vi "RedistributeArmPathPoints.vi"(1 "Desired Point Spacing (in)":dbl, 2 "Path Length (in)":dbl, 3 "ArmPathIn":T1[](array[typedef]), 4 "IndexedPathLength":dbl[](array[numeric])) -> (0 "ArmPathOut":T1[](array[typedef]))   [LabVIEW 2018]
uses:
  TypeDefs/ArmCoordinate.ctl
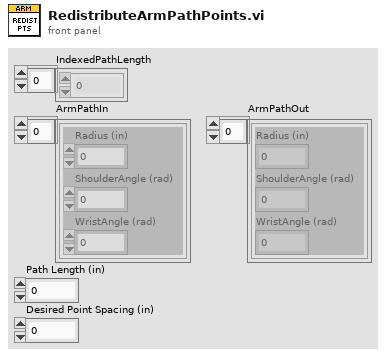
[diagram p1: front panel]
types:
  T1 = typedef "ArmCoordinate.ctl" = cluster{"Radius (in)":dbl, "ShoulderAngle (rad)":dbl, "WristAngle (rad)":dbl}
  T2 = typedef "ArmAbsolutePosition.ctl" = cluster{"X (in)":dbl, "Y (in)":dbl, "Wrist (rad)":dbl}
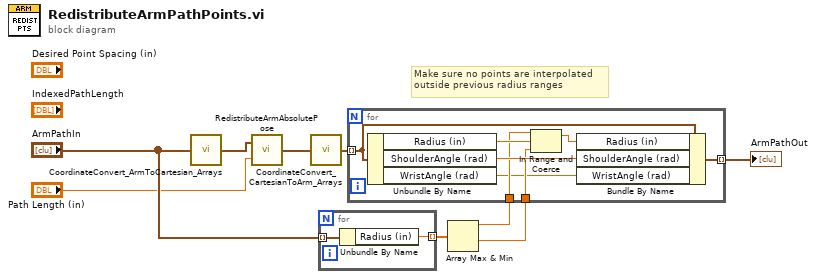
[diagram p0: block diagram]
diagram:
  # "Make sure no points are interpolated\noutside previous radius ranges"
  n1 = call "CoordinateConvert_ArmToCartesian_Arrays.vi"("ArmCoordinates"="ArmPathIn") -> ("XYPoints"=w1:T2[])
  n2 = call "RedistributeArmAbsolutePose.vi"("DesiredPointSpacing (in)"="Path Length (in)", "OriginalPoints"=w1) -> ("RedistributedPoints"=w3:T2[])
  n3 = call "CoordinateConvert_CartesianToArm_Arrays.vi"("XYPoints"=w3) -> ("ArmCoordinates"=w7:T1[])
  n4 = for {
    tunnel: "ArmPathIn" -> [w11] mode=indexing
    tunnel: [w10] -> w9 mode=indexing
    n5 = Unbundle By Name(w11) -> ("Radius (in)"=w10:dbl)
  }
  n6 = Array Max & Min(array=w9) -> (max value=w5:dbl, min value=w4:dbl)  [unwired: 2 out]
  n7 = for {
    tunnel: w7 -> [w18] mode=indexing
    tunnel: [w19] -> w6 mode=indexing
    tunnel: w5 -> [w14]
    tunnel: w4 -> [w13]
    n8 = Unbundle By Name(w18) -> ("Radius (in)"=w15:dbl, "ShoulderAngle (rad)"=w17:dbl, "WristAngle (rad)"=w12:dbl)
    n9 = In Range and Coerce(upper limit=w14, x=w15, lower limit=w13) -> (coerced(x)=w16:dbl)  [unwired: 1 out]
    n10 = Bundle By Name(cluster=w18, "Radius (in)"=w16, "ShoulderAngle (rad)"=w17, "WristAngle (rad)"=w12) -> (w19:T1)
  }
  "ArmPathOut" <- w6
